vi "Send command Get Port.vi"(8 "error in (no error)":errorcluster, 9 "Puerto":string, 10 "Marca":string, 11 "Simulado in":refnum<class "Simulado.lvclass">) -> (0 "error out":errorcluster, 1 "Command":string, 2 "Expected response":string, 3 "Simulado out":refnum<class "Simulado.lvclass">)   [LabVIEW 2020, in "Simulado.lvclass"]
doc: "Se manda el comando para obtener el estatus del puerto, se escribe en el puerto serial y se lee la respuesta que de el micro."
uses:
  Simulado.lvclass
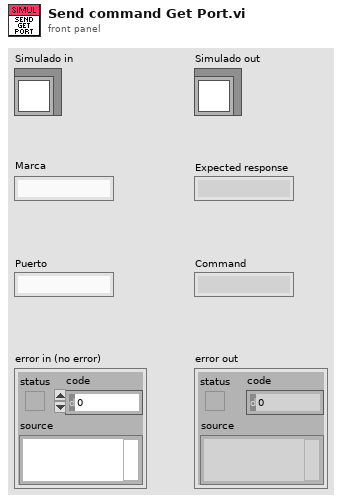
[diagram p1: front panel]
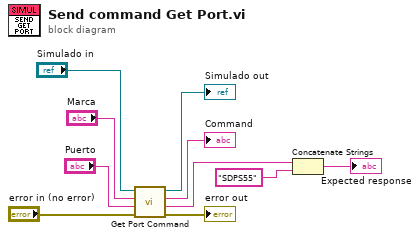
[diagram p0: block diagram]
diagram:
  n1 = call-dynamic "Get Port Command.vi"("error in (no error)"="error in (no error)", "Puerto"="Puerto", "Marca"="Marca", "Serial Device in"="Simulado in") -> ("error out"=→"error out":errorcluster, "Expected response"=w6:string, "Command"=→"Command":string, "Serial Device out"=→"Simulado out":refnum<class "Simulado.lvclass">)  [unwired: 4 in]
  n2 = Concatenate Strings(w6, "SDPS55" ("string")) -> (→"Expected response":string)
